vi "main.vi"() -> ()   [LabVIEW 2015]
uses:
  Actor/Actor.lvclass
  Actor/Type Definition/Main Ctl and VI Refenerce.ctl
  Actor/Actor.lvclass/Actor.ctl
  ImageLoad/ImageLoad.lvclass
  ImageOperaion/ImageOperation.lvclass
  FileOperation/FileOperation.lvclass
  <vilib>/Utility/miscctls.llb/LVRectTypeDef.ctl
  ImageLoad/ImageLoad.lvclass/ImageLoad.ctl
  FileOperation/FileOperation.lvclass/FileOperation.ctl
  ImageOperaion/ImageOperation.lvclass/ImageOperation.ctl
panel:
  in  "Stop":bool
  in  "Next Button":bool
  in  "Previous Button":bool
  in  "Cut":bool
  in  "Slide":i32(slide) scale=0.0..4.0
  in  "Open":bool
  out "Save Path":path
  in  "Set Size":bool
  in  "Size":cluster{"width":i16, "height":i16}={"width"=40, "height"=40}
  out "Image":T1(plugin-control)
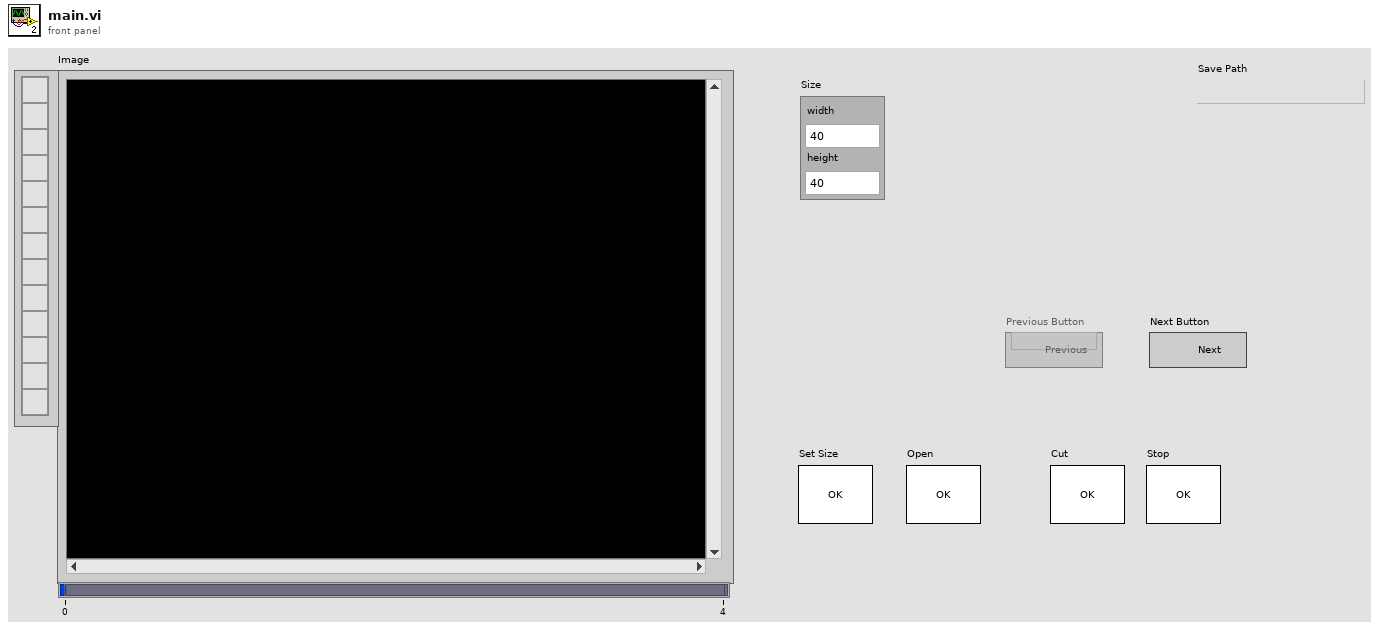
[diagram p1: front panel]
types:
  T1 = typedef "IMAQ Image.ctl" = refnum<image>
  T2 = typedef "Actor.lvclass/Main Ctl and VI Refenerce.ctl" = cluster{"Size":refnum<vi>, "Save Path":refnum<vi>, "Slide":refnum<vi>, "Cut":refnum<vi>, "Previous Button":refnum<vi>, "Next Button":refnum<vi>, "This VI":refnum<vi>}
  T3 = typedef "LVRectTypeDef.ctl" = cluster{"Left":i16, "Top":i16, "Right":i16, "Bottom":i16}
  T4 = typedef "Image Type" = u32
  T5 = typedef "ROI Descriptor" = cluster{"Global Rectangle":i32[], "Contours":cluster{"ID":enum32{"External", "Internal"}, "Type":u32, "Coordinates":i32[]}[]}
  T6 = typedef "eventvkey.ctl" = enum16{"ASCII", "Enter", "Return", "Shift", "Ctrl", "Alt", "Cmd", "Opt", "Caps", "NumLock", "Clear", "Break", "Up", "Down", "Left", "Right", "Insert", "Delete", "Home", "End", "PageUp", "PageDown", "Escape", "Help", "Pause", "ScrollLock", "F1", "F2", "F3", "F4", "F5", "F6", "F7", "F8", "F9", "F10", "F11", "F12", "F13", "F14", "F15", "F16", "F17", "F18", "F19", "F20", "F21", "F22", "F23", "F24", "Play", "VolumeUp", "VolumeDown", "Mute", "Two Byte Char"}
  T7 = enum8{"Enabled", "Disabled", "Disabled and Grayed Out"}
  T8 = cluster{"Global Rectangle":i32[], "Contours":cluster{"Contour Type":u32, "ROI Type":u32, "Points":i32[]}[]}
  T9 = typedef "IMAQ Rectangle" = cluster{"Left":i32, "Top":i32, "Right":i32, "Bottom":i32, "Rotation":dbl}
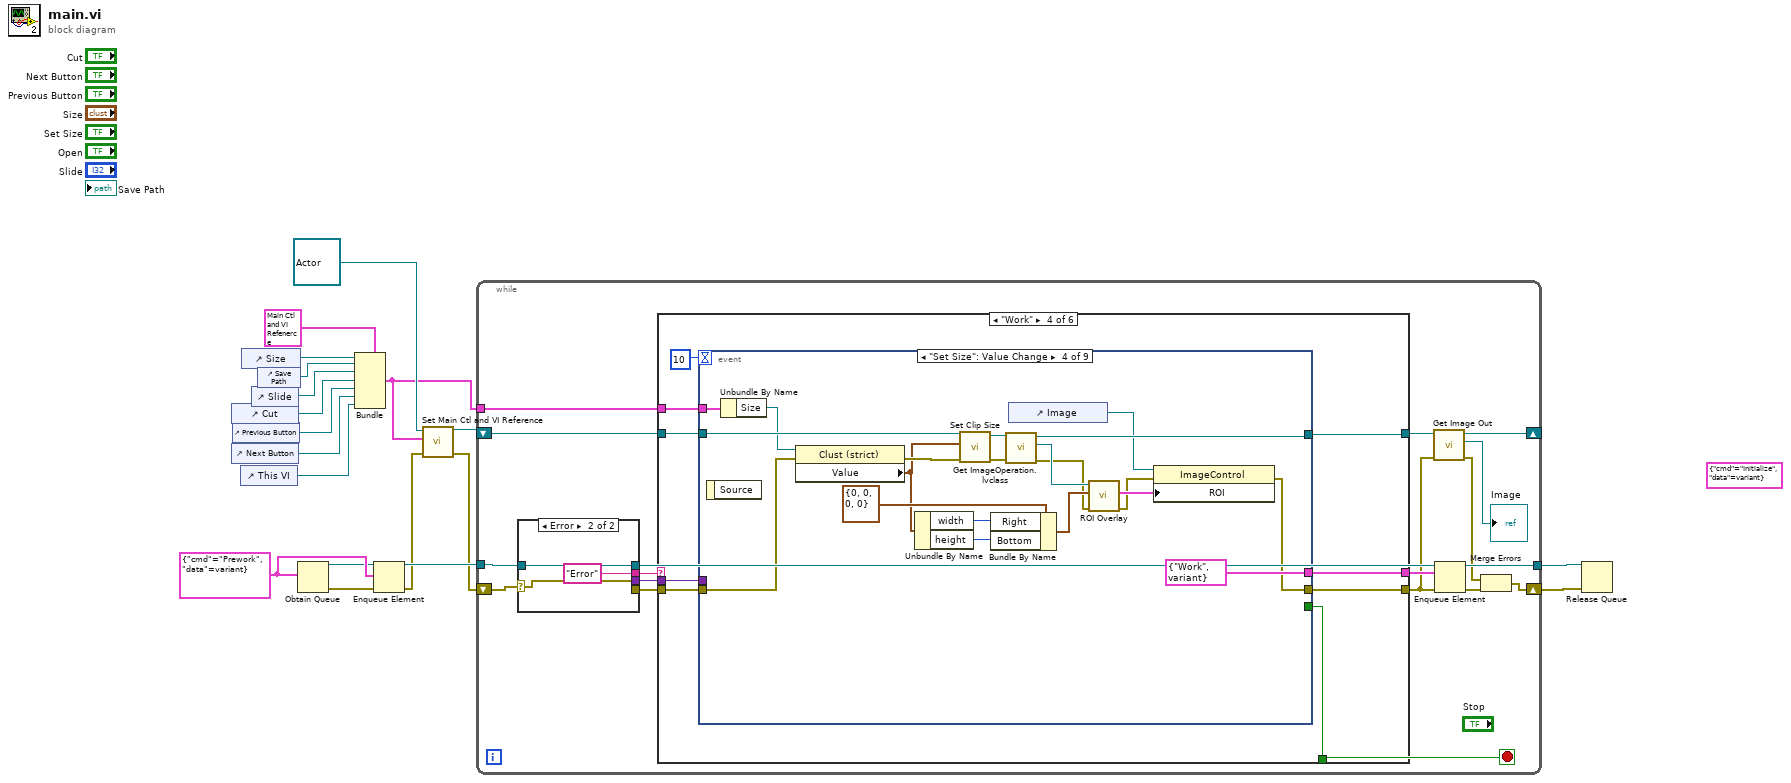
[diagram p0: block diagram]
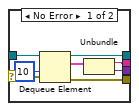
[diagram p2: hidden frame]
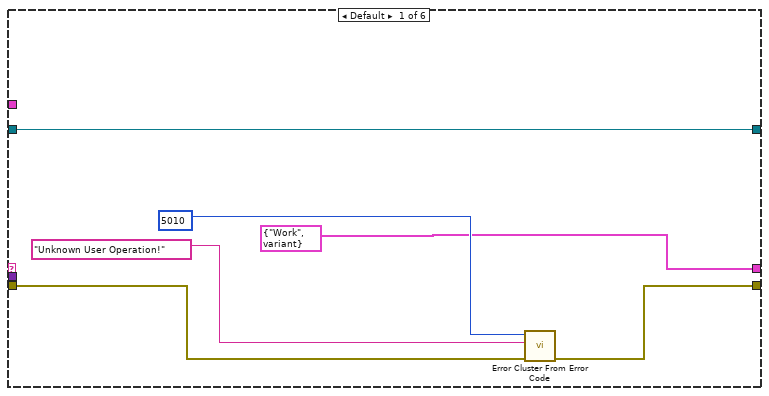
[diagram p3: hidden frame]
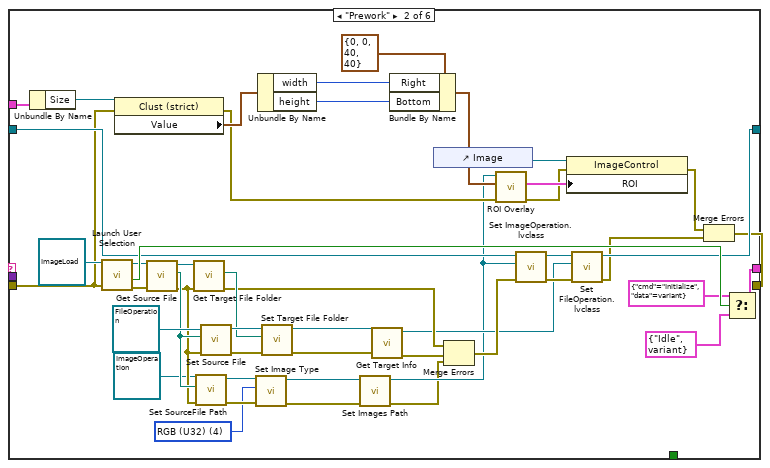
[diagram p4: hidden frame]
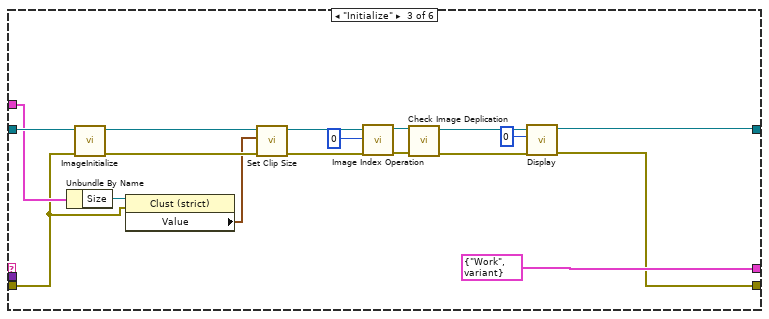
[diagram p5: hidden frame]
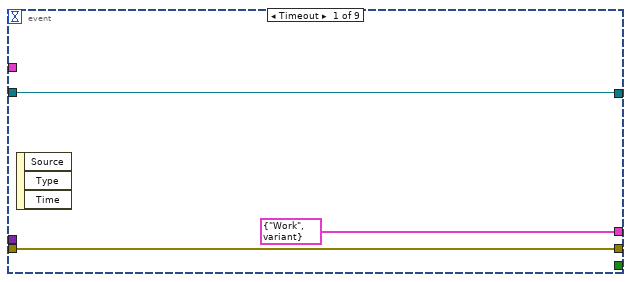
[diagram p6: hidden frame]
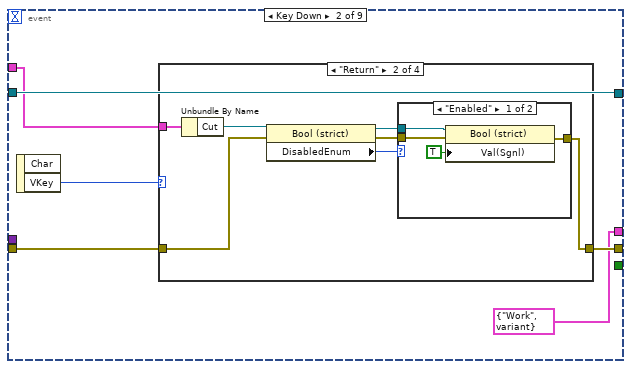
[diagram p7: hidden frame]
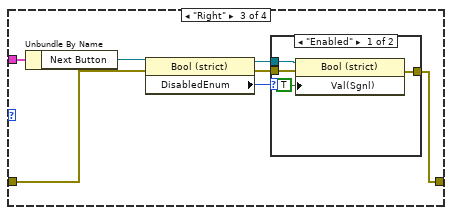
[diagram p10: hidden frame]
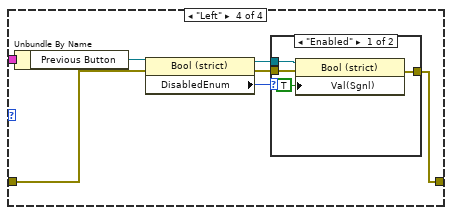
[diagram p12: hidden frame]
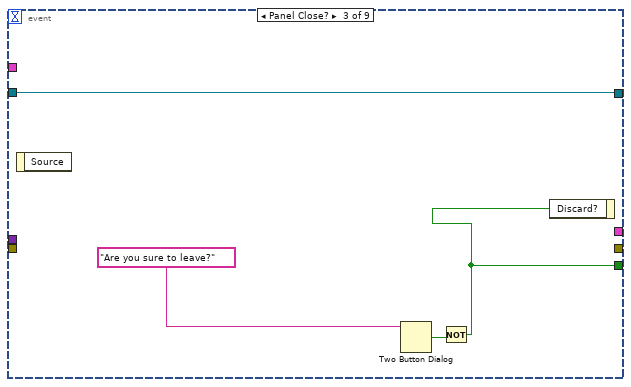
[diagram p14: hidden frame]
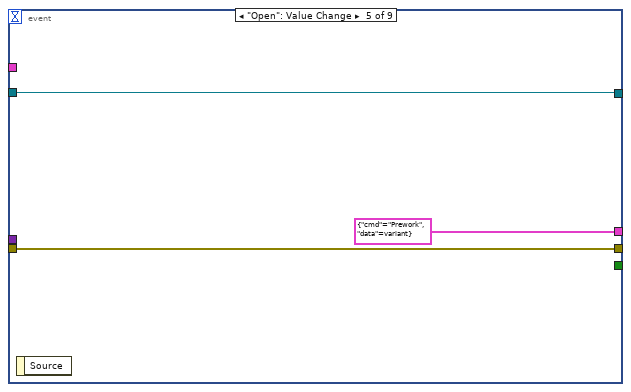
[diagram p15: hidden frame]
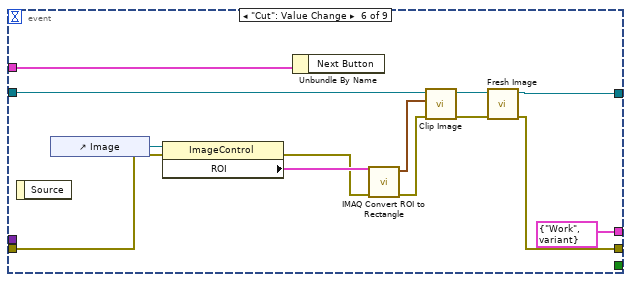
[diagram p16: hidden frame]
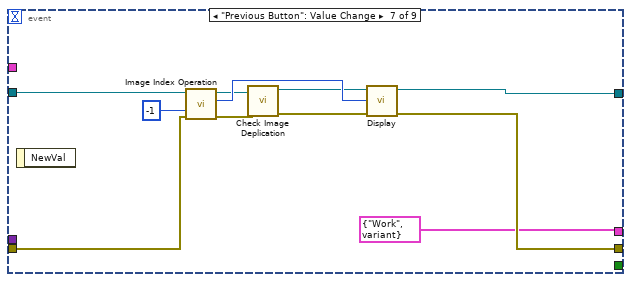
[diagram p17: hidden frame]
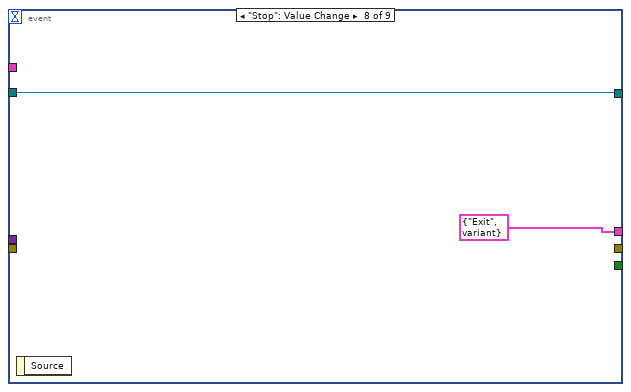
[diagram p18: hidden frame]
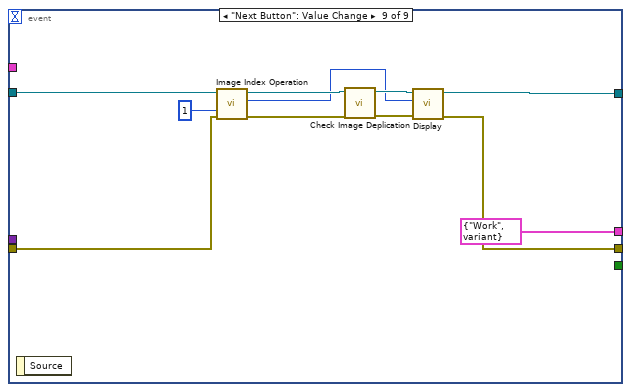
[diagram p19: hidden frame]
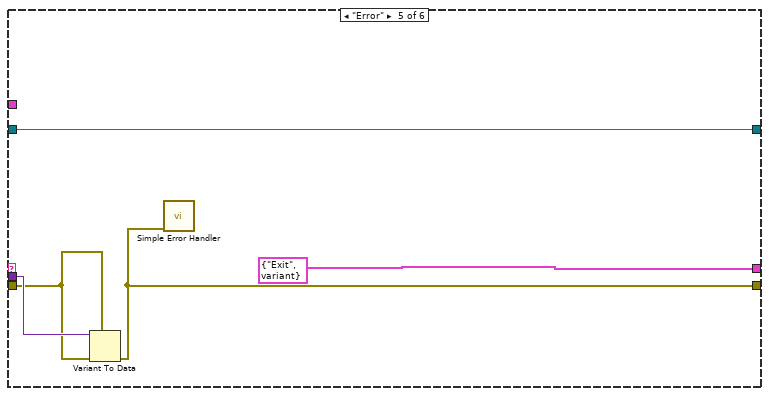
[diagram p20: hidden frame]
diagram:
  (unwired) cluster{"cmd":string, "data":variant} {"cmd"="Initialize", "data"=variant}
  w17 = cluster{"cmd":string, "data":variant} {"cmd"="Prework", "data"=variant}
  n1 = control-ref of="Cut"() -> (w4:refnum<vi>)
  n2 = control-ref of="Next Button"() -> (w2:refnum<vi>)
  n3 = control-ref of="Previous Button"() -> (w3:refnum<vi>)
  n4 = control-ref of="This VI"() -> (w1:refnum<vi>)
  n5 = control-ref of="Size"() -> (w13:refnum<vi>)
  n6 = control-ref of="Slide"() -> (w11:refnum<vi>)
  n7 = control-ref of="Save Path"() -> (w12:refnum<vi>)
  n8 = Obtain Queue(element data type=w17) -> (queue out=w14:refnum<queue>, error out=w15:errorcluster)  [unwired: 4 in, 1 out]
  n9 = Bundle(cluster=T2 {"Size"=refnum, "Save Path"=refnum, "Slide"=refnum, "Cut"=refnum, "Previous Button"=refnum, "Next Button"=refnum, "This VI"=refnum} ("Main Ctl and VI Refenerence"), "Size"=w13, "Save Path"=w12, "Slide"=w11, "Cut"=w4, "Previous Button"=w3, "Next Button"=w2, "This VI"=w1) -> (w5:T2)
  n10 = Enqueue Element(queue=w14, element=w17, error in (no error)=w15) -> (queue out=w16:refnum<queue>, error out=w8:errorcluster)  [unwired: 1 in, 1 out]
  n11 = call "Set Main Ctl and VI Reference.vi"("error in (no error)"=w8, "Main Ctl and VI Refenerence"=w5, "Actor in"=refnum<class "Actor.lvclass"> refnum) -> ("error out"=w7:errorcluster, "Actor out"=w9:refnum<class "Actor.lvclass">)  [unwired: 7 in]
  n12 = while {
    tunnel: w16 -> [w36]
    tunnel: [w29] -> w18
    shift-right: [w20] -> w19
    shift-left: w7 -> [w37]
    shift-right: [w23] -> _
    shift-left: w9 -> [w28]
    tunnel: w5 -> [w27]
    stop <- w30 stop-if-true
    n13 = case shown="Error" w37 {
      selector: w37 -> [w44 w47]
      tunnel: w36 -> [w45 w48]
      tunnel: [w42 w48] -> w34
      tunnel: [w41 _] -> w32
      tunnel: [w39 "Error" ("cmd")] -> w33
      tunnel: [w38 w47] -> w35
      frame No Error {
        n14 = Dequeue Element(queue=w45, timeout in ms (-1)=10, error in (no error)=w44) -> (queue out=w42:refnum<queue>, element=w40:cluster{"cmd":string, "data":variant}, error out=w41:errorcluster)  [unwired: 1 out]
        n15 = Unbundle(w40) -> ("cmd"=w39:string, "data"=w38:variant)
      }
      frame Error {
      }
    }
    n16 = case shown="\"Work\"" w33 {
      tunnel: w35 -> [_ _ _ w128 w243 _]
      tunnel: w32 -> [w51 w82 w109 w127 w242 w247]
      tunnel: [cluster{"cmd":string, "data":variant} {"cmd"="Work", "data"=variant} w97 cluster{"cmd":string, "data":variant} {"cmd"="Work", "data"=variant} w125 cluster{"cmd":string, "data":variant} {"cmd"="Exit", "data"=variant} cluster{"cmd":string, "data":variant} {"cmd"="Prework", "data"=variant}] -> w31
      tunnel: [w52 w72 w116 w124 w240 w247] -> w25
      tunnel: [_ _ _ w123 _ TRUE] -> w30
      tunnel: w28 -> [w49 w96 w119 w122 w239 w244]
      tunnel: [w49 w86 w115 w121 w239 w244] -> w26
      tunnel: w27 -> [_ w84 w112 w120 _ _]
      frame Default {
        n17 = call <vilib>:"Error Cluster From Error Code.vi"("error in (no error)"=w51, "error message (\"\")"="Unknown User Operation!" ("error message (\"\")"), "error code (0)"=5010) -> ("error out"=w52:errorcluster)  [unwired: 6 in]
      }
      frame "Prework" {
        w67 = T4 4 items=["Grayscale (U8)", "Grayscale (I16)", "Grayscale (SGL)", "Complex (CSG)", "RGB (U32)", "HSL (U32)", "RGB (U64)", "Grayscale (U16)"] ("Image Type(U8)")
        n18 = Unbundle By Name(w84) -> ("Size"=w83:refnum<vi>)
        n19 = call "Launch User Selection.vi"("error in (no error)"=w82, "ImageLoad in"=refnum<class "ImageLoad.lvclass"> refnum ("ImageLoad.lvclass")) -> ("error out"=w95:errorcluster, "Success?(True)"=w100:bool, "ImageLoad out"=w94:refnum<class "ImageLoad.lvclass">)  [unwired: 7 in]
        n20 = property class="Clust (strict)"(reference=w83, error in=w82) -> (error out=w66:errorcluster, "Value"=w80:cluster{"width":i16, "height":i16})  [unwired: 1 out]
        n21 = call "Get Source File.vi"("error in (no error)"=w95, "ImageLoad in"=w94) -> ("error out"=w71:errorcluster, "Source File"=w88:path, "ImageLoad out"=w93:refnum<class "ImageLoad.lvclass">)  [unwired: 7 in]
        n22 = call "Get Target File Folder.vi"("error in (no error)"=w71, "ImageLoad in"=w93) -> ("error out"=w63:errorcluster, "Target File Folder"=w90:path)  [unwired: 7 in, 1 out]
        n23 = call "Set SourceFile Path.vi"("error in (no error)"=w71, "SourceFile Path"=w88, "ImageOperation in"=refnum<class "ImageOperation.lvclass"> refnum ("ImageOperation.lvclass")) -> ("error out"=w68:errorcluster, "ImageOperation out"=w69:refnum<class "ImageOperation.lvclass">)  [unwired: 7 in]
        n24 = call "Set Source File.vi"("error in (no error)"=w71, "Source File"=w88, "FileOperation in"=refnum<class "FileOperation.lvclass"> refnum) -> ("error out"=w89:errorcluster, "FileOperation out"=w91:refnum<class "FileOperation.lvclass">)  [unwired: 7 in]
        n25 = call "Set Image Type.vi"("error in (no error)"=w68, "Image Type(U8)"=w67, "ImageOperation in"=w69) -> ("error out"=w61:errorcluster, "ImageOperation out"=w62:refnum<class "ImageOperation.lvclass">)  [unwired: 7 in]
        n26 = Unbundle By Name(w80) -> ("width"=w79:i16, "height"=w78:i16)
        n27 = call "Set Target File Folder.vi"("error in (no error)"=w89, "Target File Folder"=w90, "FileOperation in"=w91) -> ("error out"=w59:errorcluster, "FileOperation out"=w60:refnum<class "FileOperation.lvclass">)  [unwired: 7 in]
        n28 = call "Set Images Path.vi"("error in (no error)"=w61, "ImageOperation in"=w62) -> ("error out"=w55:errorcluster, "ImageOperation out"=w57:refnum<class "ImageOperation.lvclass">)  [unwired: 8 in]
        n29 = call "Get Target Info.vi"("error in (no error)"=w59, "FileOperation in"=w60) -> ("error out"=w56:errorcluster, "FileOperation out"=w58:refnum<class "FileOperation.lvclass">)  [unwired: 8 in]
        n30 = Bundle By Name(cluster=T3 {"Left"=0, "Top"=0, "Right"=40, "Bottom"=40} ("Master Bounds Rect"), "Right"=w79, "Bottom"=w78) -> (w77:T3)
        n31 = control-ref of="Image"() -> (w76:refnum<vi>)
        n32 = Merge Errors(w63, w56, w55) -> (w64:errorcluster)
        n33 = call "ROI Overlay.vi"("error in (no error)"=w66, "Master Bounds Rect"=w77, "ImageOperation in"=w57) -> ("error out"=w65:errorcluster, "ROI Descriptor"=w75:T5)  [unwired: 6 in, 1 out]
        n34 = call "Set ImageOperation.lvclass.vi"("error in (no error)"=w64, "ImageOperation.lvclass"=w57, "Actor in"=w96) -> ("error out"=w85:errorcluster, "Actor out"=w87:refnum<class "Actor.lvclass">)  [unwired: 7 in]
        n35 = property class="ImageControl"(reference=w76, error in=w65, "ROI"=w75) -> (error out=w74:errorcluster)  [unwired: 1 out]
        n36 = call "Set FileOperation.lvclass.vi"("error in (no error)"=w85, "FileOperation.lvclass"=w58, "Actor in"=w87) -> ("error out"=w73:errorcluster, "Actor out"=w86:refnum<class "Actor.lvclass">)  [unwired: 7 in]
        n37 = Merge Errors(w74, w73) -> (w72:errorcluster)
        n38 = Select(t=cluster{"cmd":string, "data":variant} {"cmd"="Initialize", "data"=variant}, s=w100, f=cluster{"cmd":string, "data":variant} {"cmd"="Idle", "data"=variant}) -> (s? t:f=w97:cluster{"cmd":string, "data":variant})
      }
      frame "Initialize" {
        n39 = Unbundle By Name(w112) -> ("Size"=w111:refnum<vi>)
        n40 = call "ImageInitialize.vi"("error in (no error)"=w109, "Actor in"=w119) -> ("error out"=w113:errorcluster, "Actor out"=w114:refnum<class "Actor.lvclass">)  [unwired: 8 in]
        n41 = property class="Clust (strict)"(reference=w111, error in=w109) -> ("Value"=w110:cluster{"width":i16, "height":i16})  [unwired: 2 out]
        n42 = call "Set Clip Size.vi"("error in (no error)"=w113, "Clip Size"=w110, "Actor in"=w114) -> ("error out"=w105:errorcluster, "Actor out"=w106:refnum<class "Actor.lvclass">)  [unwired: 7 in]
        n43 = call "Image Index Operation.vi"("error in (no error)"=w105, "IndexOperation"=0, "Actor in"=w106) -> ("error out"=w103:errorcluster, "Actor out"=w104:refnum<class "Actor.lvclass">)  [unwired: 6 in, 1 out]
        n44 = call "Check Image Deplication.vi"("error in (no error)"=w103, "Actor in"=w104) -> ("error out"=w107:errorcluster, "Actor out"=w108:refnum<class "Actor.lvclass">)  [unwired: 8 in]
        n45 = call "Display.vi"("error in (no error)"=w107, "ImageIndex"=0, "Actor in"=w108) -> ("error out"=w116:errorcluster, "Actor out"=w115:refnum<class "Actor.lvclass">)  [unwired: 7 in]
      }
      frame "Work" {
        n46 = event shown="[3] \"Set Size\": Value Change" {
          selector: _ -> [_ _ _ _ _ _ _ _ _]
          dyn-events: _ -> [_ _ _ _ _ _ _ _ _]
          timeout: 10 -> [_ _ _ _ _ _ _ _ _]
          tunnel: w128 -> [_ _ _ _ _ _ _ _ _]
          tunnel: w127 -> [w130 w134 _ w194 w200 w212 w224 _ w235]
          tunnel: [cluster{"cmd":string, "data":variant} {"cmd"="Work", "data"=variant} cluster{"cmd":string, "data":variant} {"cmd"="Work", "data"=variant} _ cluster{"cmd":string, "data":variant} {"cmd"="Work", "data"=variant} cluster{"cmd":string, "data":variant} {"cmd"="Prework", "data"=variant} cluster{"cmd":string, "data":variant} {"cmd"="Work", "data"=variant} cluster{"cmd":string, "data":variant} {"cmd"="Work", "data"=variant} cluster{"cmd":string, "data":variant} {"cmd"="Exit", "data"=variant} cluster{"cmd":string, "data":variant} {"cmd"="Work", "data"=variant}] -> w125
          tunnel: [w130 w133 _ w179 w200 w202 w220 _ w234] -> w124
          tunnel: [_ _ w176 _ _ _ _ _ _] -> w123
          tunnel: w122 -> [w129 w137 w175 w198 w201 w210 w225 w227 w237]
          tunnel: [w129 w137 w175 w183 w201 w203 w221 w227 w236] -> w121
          tunnel: w120 -> [_ w135 _ w196 _ w206 _ _ _]
          event Timeout {
            n47 = event-data() -> ()  [unwired: 1 in, 3 out]
          }
          event Key Down {
            n48 = event-data() -> ("VKey"=w136:T6)  [unwired: 1 in, 1 out]
            n49 = case shown="\"Return\"" w136 {
              tunnel: w135 -> [_ w145 w157 w169]
              tunnel: w134 -> [w138 w143 w155 w167]
              tunnel: [w138 w139 w151 w163] -> w133
              frame "ASCII", Default {
              }
              frame "Return" {
                n50 = Unbundle By Name(w145) -> ("Cut"=w144:refnum<vi>)
                n51 = property class="Bool (strict)"(reference=w144, error in=w143) -> (reference out=w140:refnum<vi>, error out=w141:errorcluster, "DisabledEnum"=w142:T7)
                n52 = case shown="\"Enabled\"" w142 {
                  tunnel: w141 -> [w148 w150]
                  tunnel: w140 -> [w149 _]
                  tunnel: [w146 w150] -> w139
                  frame "Enabled" {
                    n53 = property class="Bool (strict)"(reference=w149, error in=w148, "Val(Sgnl)"=TRUE ("Value (Signaling)")) -> (error out=w146:errorcluster)  [unwired: 1 out]
                  }
                  frame Default {
                  }
                }
              }
              frame "Right" {
                n54 = Unbundle By Name(w157) -> ("Next Button"=w156:refnum<vi>)
                n55 = property class="Bool (strict)"(reference=w156, error in=w155) -> (reference out=w152:refnum<vi>, error out=w153:errorcluster, "DisabledEnum"=w154:T7)
                n56 = case shown="\"Enabled\"" w154 {
                  tunnel: w153 -> [w160 w162]
                  tunnel: w152 -> [w161 _]
                  tunnel: [w158 w162] -> w151
                  frame "Enabled" {
                    n57 = property class="Bool (strict)"(reference=w161, error in=w160, "Val(Sgnl)"=TRUE ("Value (Signaling)")) -> (error out=w158:errorcluster)  [unwired: 1 out]
                  }
                  frame Default {
                  }
                }
              }
              frame "Left" {
                n58 = Unbundle By Name(w169) -> ("Previous Button"=w168:refnum<vi>)
                n59 = property class="Bool (strict)"(reference=w168, error in=w167) -> (reference out=w164:refnum<vi>, error out=w165:errorcluster, "DisabledEnum"=w166:T7)
                n60 = case shown="\"Enabled\"" w166 {
                  tunnel: w165 -> [w172 w174]
                  tunnel: w164 -> [w173 _]
                  tunnel: [w170 w174] -> w163
                  frame "Enabled" {
                    n61 = property class="Bool (strict)"(reference=w173, error in=w172, "Val(Sgnl)"=TRUE ("Value (Signaling)")) -> (error out=w170:errorcluster)  [unwired: 1 out]
                  }
                  frame Default {
                  }
                }
              }
            }
          }
          event Panel Close? {
            n62 = event-data() -> ()  [unwired: 1 in, 1 out]
            n63 = Two Button Dialog(message="Are you sure to leave?") -> (T button?=w177:bool)  [unwired: 2 in]
            n64 = Not(x=w177) -> (.not. x?=w176:bool)
            n65 = event-data("Discard?"=w176) -> ()  [unwired: 1 in, 1 out]
          }
          event "Set Size": Value Change {
            n66 = event-data() -> ()  [unwired: 1 in, 1 out]
            n67 = Unbundle By Name(w196) -> ("Size"=w195:refnum<vi>)
            n68 = property class="Clust (strict)"(reference=w195, error in=w194) -> (error out=w193:errorcluster, "Value"=w188:cluster{"width":i16, "height":i16})  [unwired: 1 out]
            n69 = Unbundle By Name(w188) -> ("width"=w187:i16, "height"=w186:i16)
            n70 = call "Set Clip Size.vi"("error in (no error)"=w193, "Clip Size"=w188, "Actor in"=w198) -> ("error out"=w191:errorcluster, "Actor out"=w192:refnum<class "Actor.lvclass">)  [unwired: 7 in]
            n71 = Bundle By Name(cluster=T3 {"Left"=0, "Top"=0, "Right"=0, "Bottom"=0} ("Master Bounds Rect"), "Right"=w187, "Bottom"=w186) -> (w185:T3)
            n72 = call "Get ImageOperation.lvclass.vi"("error in (no error)"=w191, "Actor in"=w192) -> ("error out"=w184:errorcluster, "ImageOperation.lvclass"=w190:refnum<class "ImageOperation.lvclass">, "Actor out"=w183:refnum<class "Actor.lvclass">)  [unwired: 7 in]
            n73 = control-ref of="Image"() -> (w182:refnum<vi>)
            n74 = call "ROI Overlay.vi"("error in (no error)"=w184, "Master Bounds Rect"=w185, "ImageOperation in"=w190) -> ("error out"=w180:errorcluster, "ROI Descriptor"=w181:T5)  [unwired: 6 in, 1 out]
            n75 = property class="ImageControl"(reference=w182, error in=w180, "ROI"=w181) -> (error out=w179:errorcluster)  [unwired: 1 out]
          }
          event "Open": Value Change {
            n76 = event-data() -> ()  [unwired: 1 in, 1 out]
          }
          event "Cut": Value Change {
            n77 = event-data() -> ()  [unwired: 1 in, 1 out]
            n78 = control-ref of="Image"() -> (w214:refnum<vi>)
            n79 = property class="ImageControl"(reference=w214, error in=w212) -> (error out=w211:errorcluster, "ROI"=w213:T8)  [unwired: 1 out]
            n80 = Unbundle By Name(w206) -> ()  [unwired: 1 out]
            n81 = call "IMAQ Convert ROI to Rectangle"("error in (no error)"=w211, "ROI Descriptor"=w213) -> ("error out"=w208:errorcluster, "Rectangle"=w209:T9)  [unwired: 7 in]
            n82 = call "Clip Image.vi"("error in (no error)"=w208, "ROI"=w209, "Actor in"=w210) -> ("error out"=w204:errorcluster, "Actor out"=w205:refnum<class "Actor.lvclass">)  [unwired: 7 in]
            n83 = call "Fresh Image.vi"("error in (no error)"=w204, "Actor in"=w205) -> ("error out"=w202:errorcluster, "Actor out"=w203:refnum<class "Actor.lvclass">)  [unwired: 8 in]
          }
          event "Previous Button": Value Change {
            n84 = event-data() -> ()  [unwired: 1 in, 1 out]
            n85 = call "Image Index Operation.vi"("error in (no error)"=w224, "IndexOperation"=-1, "Actor in"=w225) -> ("error out"=w217:errorcluster, "Index Out"=w222:i32, "Actor out"=w218:refnum<class "Actor.lvclass">)  [unwired: 6 in]
            n86 = call "Check Image Deplication.vi"("error in (no error)"=w217, "Actor in"=w218) -> ("error out"=w215:errorcluster, "Actor out"=w216:refnum<class "Actor.lvclass">)  [unwired: 8 in]
            n87 = call "Display.vi"("error in (no error)"=w215, "ImageIndex"=w222, "Actor in"=w216) -> ("error out"=w220:errorcluster, "Actor out"=w221:refnum<class "Actor.lvclass">)  [unwired: 7 in]
          }
          event "Stop": Value Change {
            n88 = event-data() -> ()  [unwired: 1 in, 1 out]
          }
          event "Next Button": Value Change {
            n89 = event-data() -> ()  [unwired: 1 in, 1 out]
            n90 = call "Image Index Operation.vi"("error in (no error)"=w235, "IndexOperation"=1, "Actor in"=w237) -> ("error out"=w231:errorcluster, "Index Out"=w228:i32, "Actor out"=w232:refnum<class "Actor.lvclass">)  [unwired: 6 in]
            n91 = call "Check Image Deplication.vi"("error in (no error)"=w231, "Actor in"=w232) -> ("error out"=w229:errorcluster, "Actor out"=w230:refnum<class "Actor.lvclass">)  [unwired: 8 in]
            n92 = call "Display.vi"("error in (no error)"=w229, "ImageIndex"=w228, "Actor in"=w230) -> ("error out"=w234:errorcluster, "Actor out"=w236:refnum<class "Actor.lvclass">)  [unwired: 7 in]
          }
        }
      }
      frame "Error" {
        n93 = Variant To Data(error in=w242, type=w242, Variant=w243) -> (error out=w240:errorcluster)  [unwired: 1 out]
        n94 = call <vilib>:"Simple Error Handler.vi"("error in (no error)"=w240) -> ()  [unwired: 4 in, 5 out]
      }
      frame "Exit" {
      }
    }
    n95 = call "Get Image Out.vi"("error in (no error)"=w25, "Actor in"=w26) -> ("error out"=w21:errorcluster, "Image"=→"Image":T1, "Actor out"=w23:refnum<class "Actor.lvclass">)  [unwired: 7 in]
    n96 = Enqueue Element(queue=w34, element=w31, error in (no error)=w25) -> (queue out=w29:refnum<queue>, error out=w22:errorcluster)  [unwired: 1 in, 1 out]
    n97 = Merge Errors(w21, w22) -> (w20:errorcluster)
  }
  n98 = Release Queue(queue=w18, error in (no error)=w19) -> ()  [unwired: 1 in, 3 out]
